vi "AOTFSetPosition.vi"   [LabVIEW 2009]
uses:
  AO Update Channel (scaled value).vi
types:
  T1 = typedef "AnalogSettings.ctt" = cluster{"PCI 671x Device Number":u32, "Samples per Unit":u32}
  T2 = typedef "AOTFSettings.ctt" = cluster{"Laser 1 Output Channel":tag, "AOTF  1 Output Voltage":dbl, "Laser 2 Output Channel":tag, "AOTF  2 Output Voltage":dbl, "Laser 3 Output Channel":tag, "AOTF  3 Output Voltage":dbl, "Pixel per Cycle":u16, "Time per Cycle  / ms":dbl, "Laser 4 Output Channel":tag, "AOTF  4 Output Voltage":dbl}
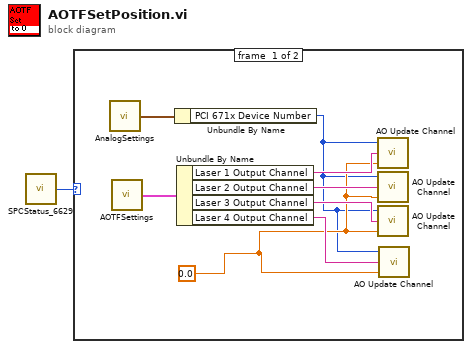
[diagram p0: block diagram]
diagram:
  n1 = call "SPCStatus_6629.vi"() -> ("Status (output)"=w1:enum16{"offline", "online", "busy"})  [unwired: 2 in]
  n2 = case shown="\"online\"" w1 {
    frame #0 {
      w3 = sgl 0.0 ("value")
      n3 = call "AnalogSettings.vi"() -> ("Analog Settings (output)"=w5:T1)  [unwired: 2 in]
      n4 = call "AOTFSettings.vi"() -> ("AOTF Setting (Output)"=w9:T2)  [unwired: 2 in]
      n5 = Unbundle By Name(w5) -> ("PCI 671x Device Number"=w2:u32)
      n6 = Unbundle By Name(w9) -> ("Laser 1 Output Channel"=w7:tag, "Laser 2 Output Channel"=w8:tag, "Laser 3 Output Channel"=w6:tag, "Laser 4 Output Channel"=w4:tag)
      n7 = call-poly "AO Update Channel.vi"("value"=w3, "channel (0)"=w7, "device"=w2) -> ()
      n8 = call-poly "AO Update Channel.vi"("value"=w3, "channel (0)"=w8, "device"=w2) -> ()
      n9 = call-poly "AO Update Channel.vi"("value"=w3, "channel (0)"=w6, "device"=w2) -> ()
      n10 = call-poly "AO Update Channel.vi"("value"=w3, "channel (0)"=w4, "device"=w2) -> ()
    }
    frame #1 {
    }
  }
